vi "TCP Read All.vi"(7 "Function Timeout":u32=1000, 8 "error in":errorcluster, 9 "TCP Timeout":i32=100, 10 "Bytes Per Loop":i32=10000, 11 "connection ID in":refnum<k5>) -> (0 "error out":errorcluster, 2 "data out":string, 3 "connection ID out":refnum<k5>)   [LabVIEW 2014]
doc: "This VI will read an XML-RPC formatted message from a TCP/IP connection. It first reads until it finds the Content-Length field in the message header and then reads the rest of the message using the Content-Length to know when the entire message has been read."
uses:
  <vilib>/Utility/error.llb/DialogType.ctl
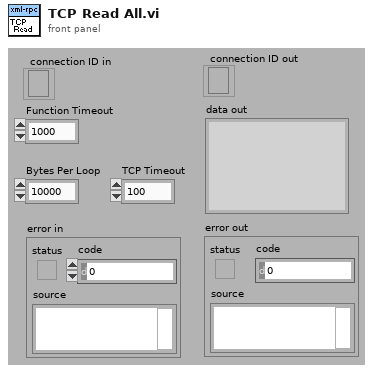
[diagram p1: front panel]
types:
  T1 = enum16{"Standard", "Buffered", "CRLF", "Immediate"}
  T2 = typedef "DialogType.ctl" = u16
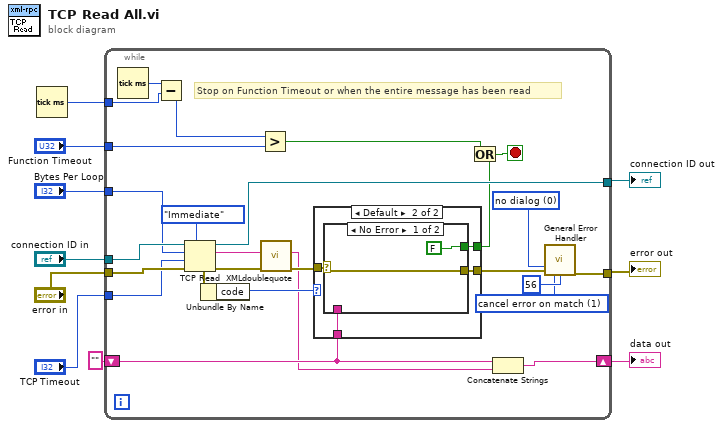
[diagram p0: block diagram]
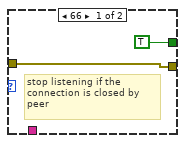
[diagram p2: hidden frame]
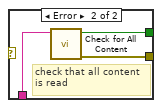
[diagram p3: hidden frame]
diagram:
  n1 = Tick Count (ms)() -> (millisecond timer value=w1:u32)
  n2 = while {
    tunnel: "error in" -> [w35]
    tunnel: "connection ID in" -> [w34]
    shift-right: [w32] -> w9
    shift-left: "" -> [w25]
    tunnel: [w31] -> w8
    tunnel: "Bytes Per Loop" -> [w28]
    tunnel: "TCP Timeout" -> [w27]
    tunnel: [w26] -> w3
    tunnel: "Function Timeout" -> [w21]
    tunnel: w1 -> [w23]
    stop <- w19 stop-if-true
    w16 = T2 0 items=["no dialog", "OK message", "continue or stop message", "OK message + warnings", "continue/stop + warnings"] ("type of dialog (OK msg:1)")
    w29 = 1 items=["no exception", "cancel error on match", "set error on match"] ("[exception action] (none:0)")
    # "Stop on Function Timeout or when the entire message has been read"
    n3 = Tick Count (ms)() -> (millisecond timer value=w24:u32)
    n4 = Subtract(x=w24, y=w23) -> (x-y=w22:u32)
    n5 = TCP Read(connection ID=w34, bytes to read=w28, error in (no error)=w35, 7:T1."Immediate" ("mode (standard)"), 9:w27) -> (connection ID out=w26:refnum<k5>, data out=w14:string, error out=w13:errorcluster)
    n6 = Unbundle By Name(w13) -> ("code"=w15:i32)
    n7 = Greater?(x=w22, y=w21) -> (0:w18:bool)
    n8 = call "XMLdoublequote.vi"("error in (no error)"=w13, "XML Input"=w14) -> ("error out"=w12:errorcluster, "XML Output"=w11:string)  [unwired: 8 in]
    n9 = case shown="Default" w15 {
      tunnel: w25 -> [_ w41]
      tunnel: [TRUE ("all content read") w40] -> w20
      tunnel: [w37 w39] -> w17
      tunnel: w12 -> [w37 w38]
      frame 66 {
        # "stop listening if the connection is closed by peer"
      }
      frame Default {
        n10 = case shown="No Error" w38 {
          selector: w38 -> [w42 _]
          tunnel: w41 -> [_ w46]
          tunnel: [FALSE ("all content read") w45] -> w40
          tunnel: [w42 w44] -> w39
          frame No Error {
          }
          frame Error {
            # "check that all content\nis read"
            n11 = call "Check for All Content.vi"("data in"=w46) -> ("error out"=w44:errorcluster, "all content read"=w45:bool)  [unwired: 9 in]
          }
        }
      }
    }
    n12 = Or(x=w18, y=w20) -> (x .or. y?=w19:bool)
    n13 = Concatenate Strings(w25, w11) -> (w32:string)
    n14 = call <vilib>:"General Error Handler.vi"("type of dialog (OK msg:1)"=w16, "error in (no error)"=w17, "[exception action] (none:0)"=w29, "[exception code]"=56) -> ("error out"=w31:errorcluster)  [unwired: 7 in, 4 out]
  }
  "error out" <- w8
  "data out" <- w9
  "connection ID out" <- w3
